vi "example test.vi"() -> ()   [LabVIEW 2013, in "EthernetIP tests.lvlib"]
uses:
  EthernetIP tests.lvlib
  configuration/EIP Tags Configuration.lvclass
  execution/EIP Tags Runtime.lvclass
  configuration/eip tag types.ctl
  <vilib>/NI/Tag Bus/dictionary/data dictionary.lvclass/data dictionary.ctl
  <vilib>/NI/Tag Bus/dictionary/lookup polymorphs/locate U16.vi
  <vilib>/NI/Tag Bus/table/data polymorphs/write one/write U16.vi
  <vilib>/NI/Tag Bus/table/data polymorphs/read one/read U16.vi
  <vilib>/NI/Tag Bus/dictionary/search/find data index.vi
  <vilib>/NI/Tag Bus/dictionary/search/search string list.vi
  <vilib>/NI/Tag Bus/dictionary/tag not found.vi
  <vilib>/NI/Tag Bus/dictionary/data dictionary.lvclass
  <vilib>/NI/Tag Bus/table/data table.lvlib
  channel/EIP Tags Channel.lvclass
  <vilib>/NI/Configuration Framework/serializable configuration/NISE_CEF_serializable configuration.lvclass
panel:
  in  "stop":bool
  in  "value TX":u16(slide)=42 scale=0.0..16000.0
  out "value RX":u16(slide) scale=0.0..16000.0
  out "final error":errorcluster
  out "output error":errorcluster
  out "input error":errorcluster
  out "output lookup error":errorcluster
  out "no data written":bool
  out "input lookup error":errorcluster
  out "init error":errorcluster
  out "correct execution settings":bool
  out "serialization problem":errorcluster
  out "invalid configuration":errorcluster
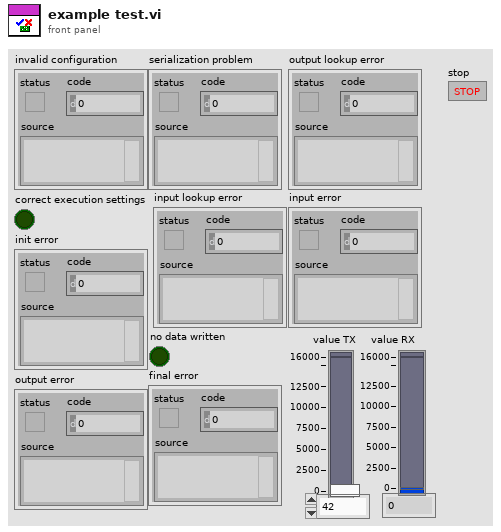
[diagram p1: front panel]
types:
  T1 = typedef "EIP Tags Configuration.lvclass/eip tag types.ctl" = enum16{"SINT", "INT", "DINT", "REAL", "BOOL", "STRING"}
  T2 = typedef "TBM channel.lvclass/data tables.ctl" = cluster{"input data":T3, "processing parameter":T3, "processing result":T3, "output data":T3}
  T3 = typedef "tag bus.lvlib/dictionary table pair.ctl" = cluster{"data dictionary":refnum<class "data dictionary.lvclass">, "data table":T4}
  T4 = typedef "tag bus.lvlib/data table.lvlib/data table.ctl" = cluster{"Double":dbl[], "Single":sgl[], "I64":i64[], "I32":i32[], "I16":i16[], "I8":i8[], "U64":u64[], "U32":u32[], "U16":u16[], "U8":u8[], "Boolean":bool[], "String":string[], "Array of Double":cluster{"DBL Array":dbl[]}[], "Array of Single":cluster{"SGL Array":sgl[]}[], "Array of I64":cluster{"I64 Array":i64[]}[], "Array of I32":cluster{"I32 Array":i32[]}[], "Array of I16":cluster{"I16 Array":i16[]}[], "Array of I8":cluster{"I8 Array":i8[]}[], "Array of U64":cluster{"U64 Array":u64[]}[], "Array of U32":cluster{"U32 Array":u32[]}[], "Array of U16":cluster{"U16 Array":u16[]}[], "Array of U8":cluster{"U8 Array":u8[]}[], "Array of Boolean":cluster{"Boolean Array":bool[]}[], "Array of String":cluster{"String Array":string[]}[]}
  T5 = typedef "TBM module execution interface.lvclass/execution settings.ctl" = cluster{"reads inputs":bool, "processes data":bool, "writes outputs":bool}
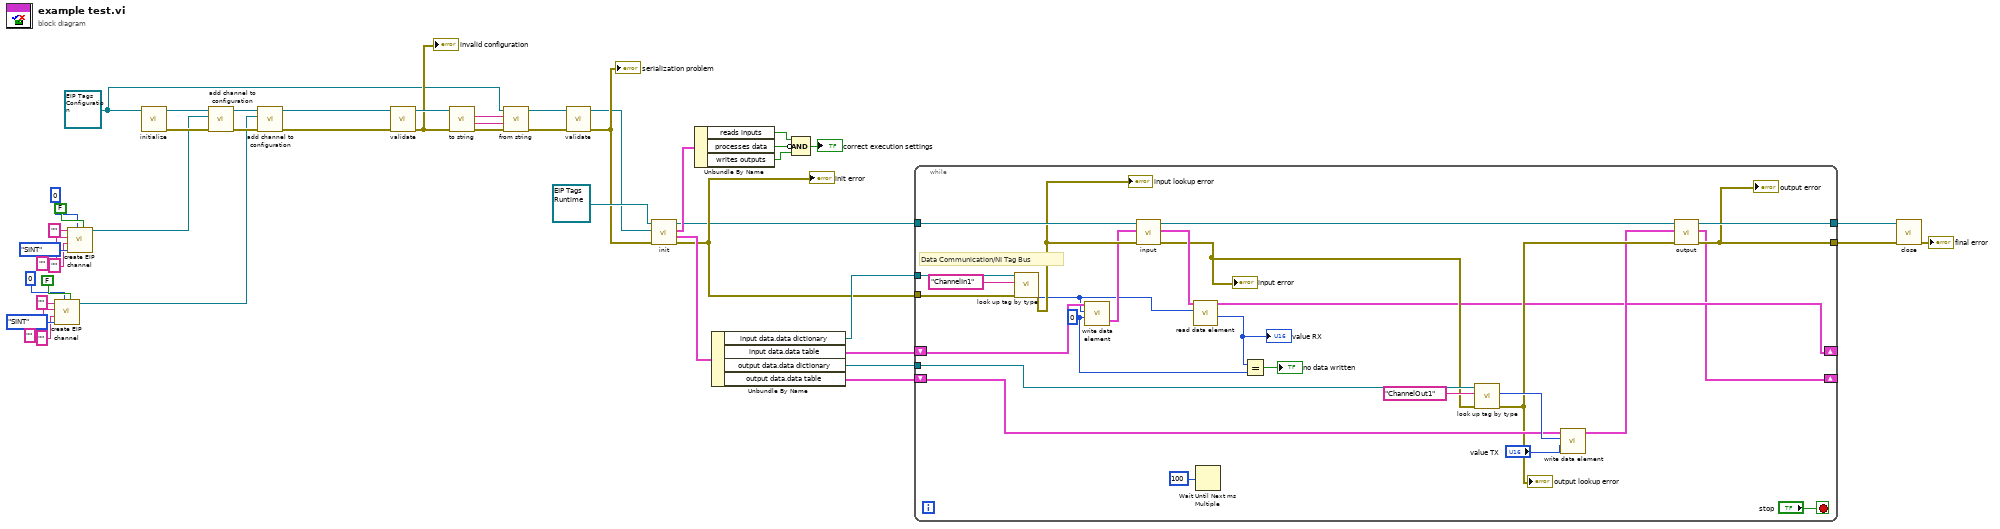
[diagram p0: block diagram]
diagram:
  w1 = refnum<class "EIP Tags Configuration.lvclass"> refnum ("tag bus configurable plugin module configuration")
  n1 = call "create EIP channel.vi"("output?"=FALSE, "element index"=0, "eip tag type"=eip_tag_types."SINT", "Tag Name"="", "Network Path"="", "name"="") -> ("EthernetIP Channel out"=w16:refnum<class "EIP Tags Channel.lvclass">)  [unwired: 5 in]
  n2 = call "create EIP channel.vi"("output?"=FALSE, "element index"=0, "eip tag type"=eip_tag_types."SINT", "Tag Name"="", "Network Path"="", "name"="") -> ("EthernetIP Channel out"=w15:refnum<class "EIP Tags Channel.lvclass">)  [unwired: 5 in]
  n3 = call <vilib>:"initialize.vi"("configuration in"=w1) -> ("error out"=w18:errorcluster, "configuration out"=w19:refnum<class "EIP Tags Configuration.lvclass">)  [unwired: 8 in, 1 out]
  n4 = call "add channel to configuration.vi"("error in"=w18, "TBM channel in"=w15, "EthernetIP configuration in"=w19) -> ("error out"=w20:errorcluster, "EthernetIP configuration out"=w21:refnum<class "EIP Tags Configuration.lvclass">)  [unwired: 7 in]
  n5 = call "add channel to configuration.vi"("error in"=w20, "TBM channel in"=w16, "EthernetIP configuration in"=w21) -> ("error out"=w17:errorcluster, "EthernetIP configuration out"=w14:refnum<class "EIP Tags Configuration.lvclass">)  [unwired: 7 in]
  n6 = call-dynamic "validate.vi"("error in"=w17, "EthernetIP configuration in"=w14) -> ("error out"=w45:errorcluster, "EthernetIP configuration out"=w46:refnum<class "EIP Tags Configuration.lvclass">)  [unwired: 8 in]
  "invalid configuration" <- w45
  n7 = call-dynamic "to string.vi"("error in"=w45, "EthernetIP configuration in"=w46) -> ("error out"=w42:errorcluster, "data"=w43:string, "version"=w44:string)  [unwired: 6 in, 1 out]
  n8 = call-dynamic "from string.vi"("error in"=w42, "data"=w43, "version"=w44, "EthernetIP configuration in"=w1) -> ("error out"=w40:errorcluster, "EthernetIP configuration out"=w41:refnum<class "EIP Tags Configuration.lvclass">)  [unwired: 6 in]
  n9 = call-dynamic "validate.vi"("error in"=w40, "EthernetIP configuration in"=w41) -> ("error out"=w38:errorcluster, "EthernetIP configuration out"=w37:refnum<class "EIP Tags Configuration.lvclass">)  [unwired: 8 in]
  "serialization problem" <- w38
  n10 = call-dynamic "init.vi"("error in"=w38, "TBM module configuration in"=w37, "EIP Tags Runtime in"=refnum<class "EIP Tags Runtime.lvclass"> refnum ("tag bus configurable plugin module")) -> ("error out"=w29:errorcluster, "data allocations"=w31:T2, "execution settings"=w36:T5, "EIP Tags Runtime out"=w27:refnum<class "EIP Tags Runtime.lvclass">)  [unwired: 5 in]
  "init error" <- w29
  n11 = Unbundle By Name(w36) -> ("reads inputs"=w33:bool, "processes data"=w35:bool, "writes outputs"=w34:bool)
  n12 = Unbundle By Name(w31) -> ("input data.data dictionary"=w30:refnum<class "data dictionary.lvclass">, "input data.data table"=w28:T4, "output data.data dictionary"=w26:refnum<class "data dictionary.lvclass">, "output data.data table"=w25:T4)
  n13 = Compound Arithmetic op=AND(w33, invert w35, w34) -> (→"correct execution settings":bool)
  n14 = while {
    tunnel: w30 -> [w73]
    tunnel: w29 -> [w72]
    tunnel: w27 -> [w69]
    tunnel: w26 -> [w62]
    tunnel: [w53] -> w24
    tunnel: [w52] -> w23
    shift-right: [w49] -> _
    shift-left: w25 -> [w59]
    shift-right: [w50] -> _
    shift-left: w28 -> [w70]
    stop <- "stop" stop-if-true
    w51 = u16 0 ("value")
    # "Data Communication/NI Tag Bus"
    n15 = call-poly <vilib>:"look up tag by type.vi"("error in"=w72, "name"="ChannelIn1" ("channel name"), "data dictionary in"=w73) -> ("error out"=w68:errorcluster, "index"=w65:i32)  [unwired: 6 in, 1 out]
    "input lookup error" <- w68
    n16 = call-poly <vilib>:"write data element.vi"("value"=w51, "index"=w65, "data table in"=w70) -> ("data table out"=w67:T4)  [unwired: 8 in]
    n17 = call-dynamic "input.vi"("error in"=w68, "data table in"=w67, "EthernetIP runtime in"=w69) -> ("error out"=w58:errorcluster, "data table out"=w66:T4, "EthernetIP runtime out"=w55:refnum<class "EIP Tags Runtime.lvclass">)  [unwired: 6 in]
    "input error" <- w58
    n18 = call-poly <vilib>:"read data element.vi"("index"=w65, "data table in"=w66) -> ("value"=w64:u16, "data table out"=w50:T4)  [unwired: 8 in]
    "value RX" <- w64
    n19 = Wait Until Next ms Multiple(millisecond multiple=u32 100) -> ()  [unwired: 1 out]
    n20 = Equal?(x=w64, y=w51) -> (x = y?=→"no data written":bool)
    n21 = call-poly <vilib>:"look up tag by type.vi"("error in"=w58, "name"="ChannelOut1" ("channel name"), "data dictionary in"=w62) -> ("error out"=w56:errorcluster, "index"=w60:i32)  [unwired: 6 in, 1 out]
    "output lookup error" <- w56
    n22 = call-poly <vilib>:"write data element.vi"("value"="value TX", "index"=w60, "data table in"=w59) -> ("data table out"=w54:T4)  [unwired: 8 in]
    n23 = call-dynamic "output.vi"("error in"=w56, "data table in"=w54, "EIP Tags Runtime in"=w55) -> ("error out"=w52:errorcluster, "data table out"=w49:T4, "EIP Tags Runtime out"=w53:refnum<class "EIP Tags Runtime.lvclass">)  [unwired: 6 in]
    "output error" <- w52
  }
  n24 = call-dynamic "close.vi"("error in"=w23, "EIP Tags Runtime in"=w24) -> ("error out"=→"final error":errorcluster)  [unwired: 9 in]
